vi "Strain (Rosette) - SW-Timed Input.vi"() -> ()   [LabVIEW 2022 SP3]
doc: "This example demonstrates how to continuously acquire rosette strain gage measurements using a DAQmx device.\n\nFor instructions on how to connect your signals to the DAQ device, refer to your device documentation."
uses:
  <vilib>/Utility/error.llb/DialogType.ctl
  <vilib>/DAQmx/read.llb/DAQmx Read (Analog 1D DBL NChan 1Samp).vi
  <vilib>/DAQmx/create/channels.llb/DAQmx Create Channel (AI-Strain-Rosette Strain Gage).vi
  <vilib>/DAQmx/calibration/calibrationInfo.llb/DAQmx Perform Shunt Calibration Ex (Strain).vi
  <vilib>/DAQmx/miscellaneous.llb/DAQmx Fill In Error Info.vi
  <resource>/objmgr/daqmx.rc
panel:
  out "Acquired Data":cluster{string, "Waveform":dbl}[](array[cluster])
  in  "Loop Time (ms)":u32=100
  in  "Rosette Configuration":T1={"Rosette Type"=15968, "Gage Orientation"=0.0, "Rosette Measurements"=[15971, 15972, 15973, 15974, 15975, 15976, 15977, 15978]} {"Rosette Measurements" items=["Principal Strain 1"=15971, "Principal Strain 2"=15972, "Principal Strain Angle"=15973, "Cartesian Strain X"=15974, "Cartesian Strain Y"=15975, "Cartesian Shear Strain XY"=15976, "Maximum Shear Strain"=15977, "Maximum Shear Strain Angle"=15978]; "Rosette Type" items=["Rectangular Rosette"=15968, "Delta Rosette"=15969, "Tee Rosette"=15970]}
  in  "Strain Gage Information":T2={"Gage Factor"=2.0, "Nominal Gage Resistance"=350.0, "Poisson Ratio"=0.3} {"Nominal Gage Resistance" format="%0.2f"; "Poisson Ratio" format="%0.2f"; "Gage Factor" format="%0.2f"}
  in  "Bridge Information":T3={"Strain Configuration"=10271, "Lead Wire Resistance"=0.0, "Voltage Excitation Source"=10200, "Voltage Excitation Value"=2.5} {"Voltage Excitation Source" items=["Internal"=10200, "External"=10167, "None"=10230]; "Voltage Excitation Value" format="%0.2f"; "Lead Wire Resistance" format="%0.2f"; "Strain Configuration" items=["Full Bridge I"=10183, "Full Bridge II"=10184, "Full Bridge III"=10185, "Half Bridge I"=10188, "Half Bridge II"=10189, "Quarter Bridge I"=10271, "Quarter Bridge II"=10272]}
  in  "Do Shunt Cal?":bool
  in  "Shunt Element Location":i32(ring)=12465 caption="shunt element location" items=["R1"=12465, "R2"=12466, "R3"=12467, "R4"=14813, "None"=10230]
  in  "Shunt Resistance":dbl=100000.0 format="%#.3p"
  in  "Do Offset Null?":bool
  in  "Minimum Value":dbl=-0.001
  in  "Maximum Value":dbl=0.001
  in  "Physical Channels":tag="Dev1/ai0:2"
  in  "Stop":bool
  # "Channel Settings"
  # "Acquired Data"
  # "Shunt Calibration and Offset Null Settings"
  # "Timing Settings"
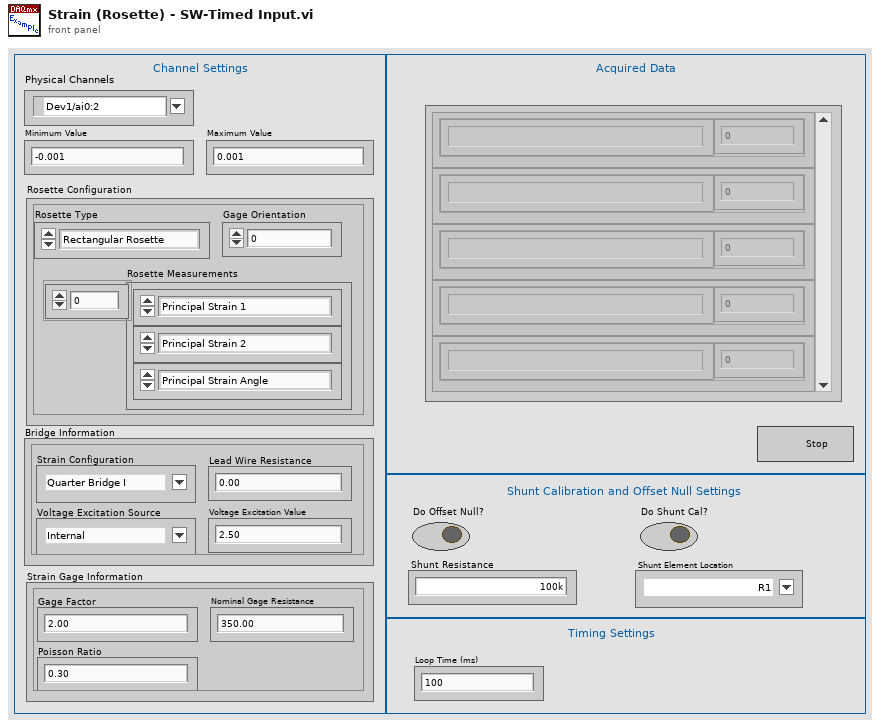
[diagram p1: front panel]
types:
  T1 = cluster{"Rosette Type":i32, "Gage Orientation":dbl, "Rosette Measurements":i32[]}
  T2 = cluster{"Gage Factor":dbl, "Nominal Gage Resistance":dbl, "Poisson Ratio":dbl}
  T3 = cluster{"Strain Configuration":i32, "Lead Wire Resistance":dbl, "Voltage Excitation Source":i32, "Voltage Excitation Value":dbl}
  T4 = typedef "DialogType.ctl" = u16
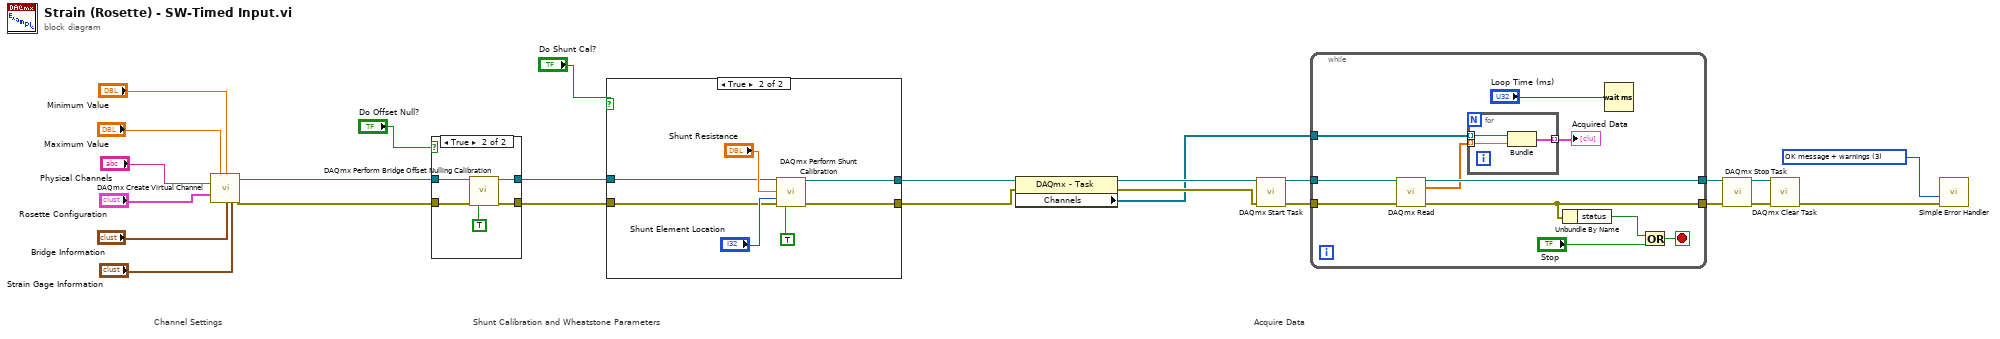
[diagram p0: block diagram]
diagram:
  w6 = T4 3 items=["no dialog", "OK message", "continue or stop message", "OK message + warnings", "continue/stop + warnings"] ("type of dialog (OK msg:1)")
  # "Acquire Data"
  # "Shunt Calibration and Wheatstone Parameters"
  # "Channel Settings"
  n1 = call-poly <vilib>:"DAQmx Create Virtual Channel.vi"("maximum value"="Maximum Value", "minimum value"="Minimum Value", "physical channels"="Physical Channels", "rosette configuration"="Rosette Configuration", "bridge information"="Bridge Information", "strain gage information"="Strain Gage Information") -> ("task out"=w12:refnum<k21>, "error out"=w11:errorcluster)  [unwired: 8 in]
  n2 = case shown="True" "Do Offset Null?" {
    tunnel: w12 -> [w27 w32]
    tunnel: w11 -> [w26 w31]
    tunnel: [w26 w28] -> w13
    tunnel: [w27 w29] -> w15
    frame False {
    }
    frame True {
      n3 = call <vilib>:"DAQmx Perform Bridge Offset Nulling Calibration.vi"("task/channels in"=w32, "error in"=w31, "skip unsupported channels"=TRUE) -> ("task out"=w29:refnum<k21>, "error out"=w28:errorcluster)  [unwired: 11 in]
    }
  }
  n4 = case shown="True" "Do Shunt Cal?" {
    tunnel: [w33 w41] -> w7
    tunnel: [w34 w40] -> w8
    tunnel: w15 -> [w34 w36]
    tunnel: w13 -> [w33 w35]
    frame False {
    }
    frame True {
      n5 = call-poly <vilib>:"DAQmx Perform Shunt Calibration.vi"("task/channels in"=w36, "shunt resistance"="Shunt Resistance", "shunt element location"="Shunt Element Location", "error in"=w35, "skip unsupported channels"=TRUE) -> ("task out"=w40:refnum<k21>, "error out"=w41:errorcluster)  [unwired: 9 in]
    }
  }
  n6 = property class="DAQmx - Task"(reference=w8, error in=w7) -> (reference out=w10:refnum<k21>, error out=w9:errorcluster, "Channels"=w1:refnum<k21>[])
  n7 = call <vilib>:"DAQmx Start Task.vi"("task/channels in"=w10, "error in"=w9) -> ("task out"=w25:refnum<k21>, "error out"=w24:errorcluster)  [unwired: 12 in]
  n8 = while {
    tunnel: w25 -> [w45]
    tunnel: w24 -> [w52]
    tunnel: [w49] -> w4
    tunnel: [w50] -> w5
    tunnel: w1 -> [w44]
    stop <- w51 stop-if-true
    n9 = call-poly <vilib>:"DAQmx Read.vi"("task/channels in"=w45, "error in"=w52) -> ("task out"=w50:refnum<k21>, "data"=w43:dbl[], "error out"=w49:errorcluster)  [unwired: 11 in]
    n10 = for {
      tunnel: [w55] -> w42 mode=indexing
      tunnel: w44 -> [w54] mode=indexing
      tunnel: w43 -> [w53] mode=indexing
      n11 = Bundle(w54, "Waveform"=w53) -> (w55:cluster{refnum<k21>, "Waveform":dbl})  [unwired: 1 in]
    }
    "Acquired Data" <- w42
    n12 = Unbundle By Name(w49) -> ("status"=w48:bool)
    n13 = Wait (ms)(milliseconds to wait="Loop Time (ms)") -> ()  [unwired: 1 out]
    n14 = Or(x=w48, y="Stop") -> (x .or. y?=w51:bool)
  }
  n15 = call <vilib>:"DAQmx Stop Task.vi"("task/channels in"=w5, "error in"=w4) -> ("task out"=w3:refnum<k21>, "error out"=w2:errorcluster)  [unwired: 12 in]
  n16 = call <vilib>:"DAQmx Clear Task.vi"("task in"=w3, "error in"=w2) -> ("error out"=w23:errorcluster)  [unwired: 13 in]
  n17 = call <vilib>:"Simple Error Handler.vi"("type of dialog (OK msg:1)"=w6, "error in (no error)"=w23) -> ()  [unwired: 3 in, 5 out]
